vi "Orca catalog parameters.vi"() -> ()   [LabVIEW 2011]
panel:
  out "H Width":T1
  out "V Width":T1
  out "Camera info":string[](array[string])
  out "Parameters":T2(array[cluster])
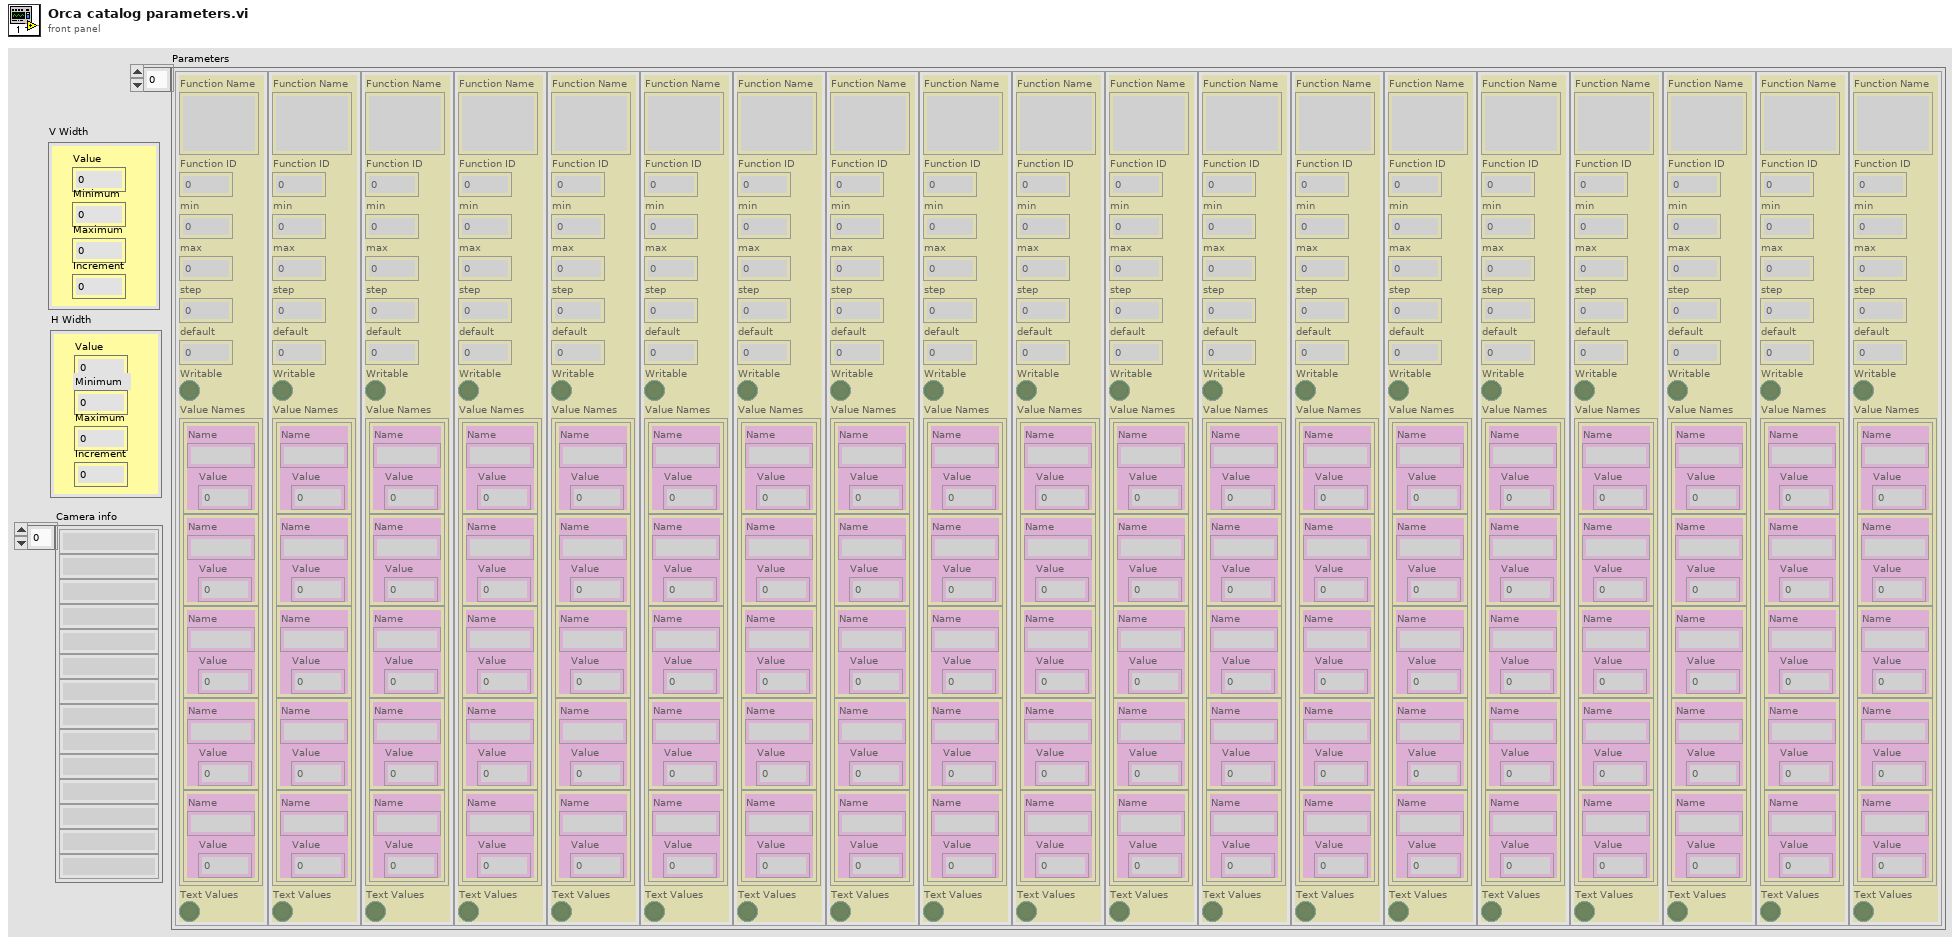
[diagram p1: front panel]
types:
  T1 = cluster{"Value":i32, "Minimum":i32, "Maximum":i32, "Increment":i32}
  T2 = cluster{"Function Name":string, "Function ID":dbl, "min":dbl, "max":dbl, "step":dbl, "default":dbl, "Writable":bool, "Value Names":cluster{"Name":string, "Value":dbl}[], "Text Values":bool}[]
  T3 = cluster{"Function Name":string, "Function ID":dbl}[]
  T4 = cluster{"Function Name":string, "Function ID":dbl, "min":dbl, "max":dbl, "step":dbl, "default":dbl, "Writable":bool, "Value Names":cluster{"Name":string, "Value":dbl}[], "Text Values":bool}
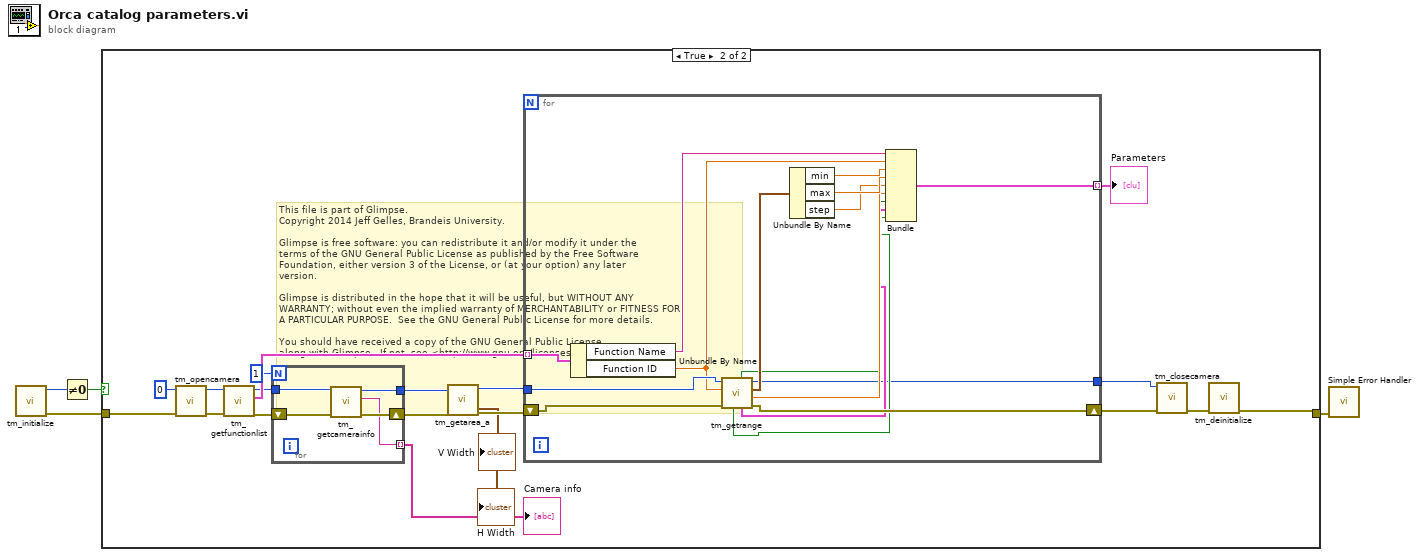
[diagram p0: block diagram]
diagram:
  # "This file is part of Glimpse. \nCopyright 2014 Jeff Gelles, Brandeis University.    \n\nGlimpse is free software: you can redistribute it and/or modify it under the \nterms of the GNU General Public License as published by the Free Software \nFoundation, either version 3 of the License, or (at your option) any later \nversion.\n\nGlimpse is distributed in the hope that it will be useful, but WITHOUT ANY \nWARRANTY; without even the implied warranty of MERCHANTABILITY or FITNESS FOR \nA PARTICULAR PURPOSE.  See the GNU General Public License for more details.\n\nYou should have received a copy of the GNU General Public License\nalong with Glimpse.  If not, see <http://www.gnu.org/licenses/>."
  n1 = call <userlib>:"tm_initialize.vi"() -> ("error out"=w2:errorcluster, "Number Of Cameras"=w4:u32)  [unwired: 10 in]
  n2 = Not Equal To 0?(x=w4) -> (x != 0?=w3:bool)
  n3 = case shown="True" w3 {
    tunnel: [w5 w16] -> w1
    tunnel: w2 -> [w5 w25]
    frame False {
    }
    frame True {
      n4 = call <userlib>:"tm_opencamera.vi"("error in (no error)"=w25, "Camera Index"=u32 0) -> ("error out"=w22:errorcluster, "Handle out"=w23:u32)  [unwired: 8 in]
      n5 = call <userlib>:"tm_getfunctionlist.vi"("error in (no error)"=w22, "Handle in"=w23) -> ("error out"=w15:errorcluster, "Function List"=w20:T3, "Handle out"=w14:u32)  [unwired: 7 in]
      n6 = for {
        N: 1 -> [_]
        tunnel: w14 -> [w28]
        tunnel: [w27] -> w9
        tunnel: [w26] -> w12 mode=indexing
        shift-right: [w29] -> w11
        shift-left: w15 -> [w30]
        n7 = call <userlib>:"tm_getcamerainfo.vi"("error in (no error)"=w30, "Handle in"=w28) -> ("error out"=w29:errorcluster, "String"=w26:string, "Handle out"=w27:u32)  [unwired: 7 in]
      }
      "Camera info" <- w12
      n8 = call <userlib>:"tm_getarea_a.vi"("error in (no error)"=w11, "Handle in"=w9) -> ("error out"=w10:errorcluster, "Handle out"=w8:u32, "H Width"=→"H Width":T1, "V Width"=→"V Width":T1)  [unwired: 4 in, 2 out]
      n9 = for {
        tunnel: w20 -> [w46] mode=indexing
        shift-right: [w44] -> w18
        shift-left: w10 -> [w45]
        tunnel: w8 -> [w43]
        tunnel: [w32] -> w19 mode=indexing
        tunnel: [w31] -> w17
        n10 = Unbundle By Name(w46) -> ("Function Name"=w42:string, "Function ID"=w41:dbl)
        n11 = call <userlib>:"tm_getrange.vi"("error in (no error)"=w45, "Parameter"=w41, "Handle in"=w43) -> ("error out"=w44:errorcluster, "default"=w36:dbl, "Range"=w40:cluster{"min":dbl, "max":dbl, "step":dbl}, "Handle out"=w31:u32, "Value Names"=w34:cluster{"Name":string, "Value":dbl}[], "Writable"=w35:bool, "Text Values"=w33:bool)  [unwired: 2 in]
        n12 = Unbundle By Name(w40) -> ("min"=w39:dbl, "max"=w38:dbl, "step"=w37:dbl)
        n13 = Bundle("Function Name"=w42, "Function ID"=w41, "min"=w39, "max"=w38, "step"=w37, "default"=w36, "Writable"=w35, "Value Names"=w34, "Text Values"=w33) -> (w32:T4)  [unwired: 1 in]
      }
      "Parameters" <- w19
      n14 = call <userlib>:"tm_closecamera.vi"("error in (no error)"=w18, "Handle in"=w17) -> ("error out"=w24:errorcluster)  [unwired: 9 in]
      n15 = call <userlib>:"tm_deinitialize.vi"("error in (no error)"=w24) -> ("error out"=w16:errorcluster)  [unwired: 10 in]
    }
  }
  n16 = call <vilib>:"Simple Error Handler.vi"("error in (no error)"=w1) -> ()  [unwired: 4 in, 5 out]
